vi "Drive.vi"(9 "Joystick 1":dbl format="%#_13g", 10 "RT":dbl format="%#_13g", 11 "LT":dbl format="%#_13g") -> ()   [LabVIEW 2016]
panel:
  out "Right":dbl format="%#_13g"
  out "Left":dbl format="%#_13g"
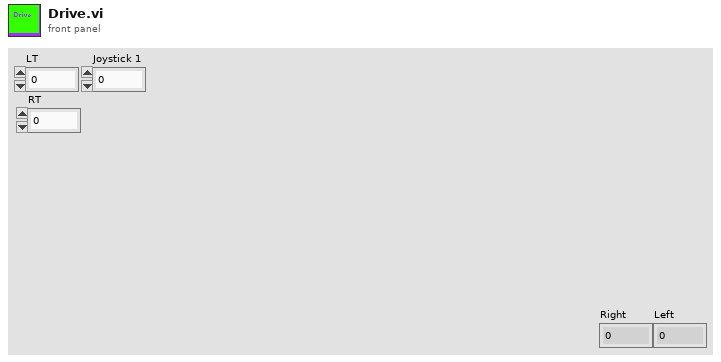
[diagram p1: front panel]
types:
  T1 = typedef "WPI_MotorControlDeviceRef.ctl" = cluster{"DeviceStatus":errorcluster, "Type":T2, "PWM":cluster{"PWM Channel":T3, "DeadBand":T4}, "CAN":cluster{"Device Number":u8, "SetOutput VI Ref":variant, "GetOutput VI Ref":variant, "Enable VI Ref":variant, "Disable VI Ref":variant, "Data":variant}, "Invert":bool}
  T2 = typedef "WPI_MotorControlType.ctl" = enum16{"PWM", "CAN"}
  T3 = typedef "FPGA_DIOPWMChannel.ctl" = enum8{"PWM 0", "PWM 1", "PWM 2", "PWM 3", "PWM 4", "PWM 5", "PWM 6", "PWM 7", "PWM 8", "PWM 9", "PWM MXP 0", "PWM MXP 1", "PWM MXP 2", "PWM MXP 3", "PWM MXP 4", "PWM MXP 5", "PWM MXP 6", "PWM MXP 7", "PWM MXP 8", "PWM MXP 9", "Invalid"}
  T4 = typedef "WPI_PWMDeadband.ctl" = cluster{"Name":string, "maxPositivePwm":i32, "minPositivePwm":i32, "centerPwm":i32, "maxNegativePwm":i32, "minNegativePwm":i32, "angularRange":u16}
  T5 = typedef "WPI_CANTalonSRX_GlobalStatus.ctl" = cluster{"Applied Throttle":dbl, "Module Enabled":bool, "CAN Error":errorcluster, "Closed Loop Error":dbl, "Forward Limit Switch Closed":bool, "Reverse Limit Switch Closed":bool, "Sensor Position":dbl, "Sensor Velocity":dbl, "Current":dbl, "Sticky Fault - Over Temp":bool, "Sticky Fault - Under Voltage":bool, "Sticky Fault - Forward Limit":bool, "Sticky Fault - Reverse Limit":bool, "Sticky Fault - Forward Soft Limit":bool, "Sticky Fault - Reverse Soft Limit":bool, "Brake is Enabled":bool, "Encoder Position":dbl, "Encoder Velocity":dbl, "Encoder Index Count":dbl, "Encoder A Pin State":bool, "Encoder B Pin State":bool, "Encoder Index Pin State":bool, "Analog In":dbl, "Analog In Velocity":dbl, "Temperature (C)":dbl, "Battery Voltage":dbl, "Control 5 Is Supported":bool, "Current Profile Slot Select":dbl, "Pos Div 8":bool, "Vel Div 4":bool, "Pulse Width Position":i32, "Pulse Width Velocity":i32, "Pulse Width Rise To Rise (us)":i32, "Pulse Width Rise To Fall (us)":i32, "Mot Prof Active Is Under Run":bool, "Mot Prof Active Has Under Run":bool, "Mot Prof Active Is Last":bool, "Mot Prof Active Velocity Only":bool, "Mot Prof Active Is Valid":bool, "Mot Prof Buffer Is Full":bool, "Mot Prof Active Profile Slot Select":i32, "Mot Prof NextID":i32, "Mot Prof Count":i32, "Mot Prof Active Velocity":dbl, "Mot Prof Active Position":dbl, "Mot Prof Output Enable":i32}
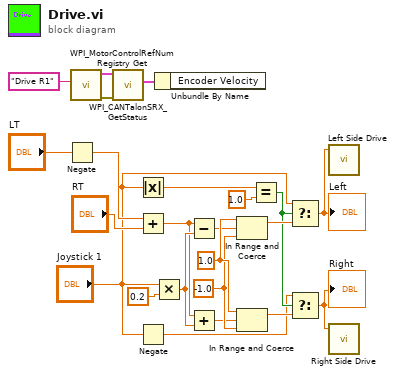
[diagram p0: block diagram]
diagram:
  w18 = -1.0 ("Numeric 4")
  w19 = 1.0 ("Numeric 4")
  n1 = Negate(x="LT") -> (-x=w17:dbl)
  n2 = call <vilib>:"WPI_MotorControlRefNum Registry Get.vi"("refnum name"="Drive R1") -> ("error out"=w22:errorcluster, "MotorControlDevRef"=w23:T1)  [unwired: 9 in]
  n3 = call <vilib>:"WPI_CANTalonSRX_GetStatus.vi"("error in (no error)"=w22, "CAN Talon SRX Ref"=w23) -> ("Talon SRX Status"=w21:T5)  [unwired: 7 in, 2 out]
  n4 = Absolute Value(x="Joystick 1") -> (abs(x)=w11:dbl)
  n5 = Add(x=w17, y="RT") -> (x+y=w14:dbl)
  n6 = Negate(x="Joystick 1") -> (-x=w6:dbl)
  n7 = Multiply(x="Joystick 1", y=0.2) -> (x*y=w15:dbl)
  n8 = Unbundle By Name(w21) -> ()  [unwired: 1 out]
  n9 = Subtract(x=w14, y=w15) -> (x-y=w12:dbl)
  n10 = Add(x=w14, y=w15) -> (x+y=w13:dbl)
  n11 = In Range and Coerce(upper limit=w19, x=w12, lower limit=w18) -> (coerced(x)=w9:dbl)  [unwired: 1 out]
  n12 = In Range and Coerce(upper limit=w19, x=w13, lower limit=w18) -> (coerced(x)=w8:dbl)  [unwired: 1 out]
  n13 = Equal?(x=w11, y=1.0) -> (x = y?=w7:bool)
  n14 = Select(t="Joystick 1", s=w7, f=w9) -> (s? t:f=w2:dbl)
  "Left" <- w2
  n15 = Select(t=w6, s=w7, f=w8) -> (s? t:f=w1:dbl)
  "Right" <- w1
  n16 = call "Left Side Drive.vi"("Effort"=w2) -> ()  [unwired: 11 in]
  n17 = call "Right Side Drive.vi"("Effort"=w1) -> ()  [unwired: 11 in]
